vi "Prj2_Main.vi"() -> ()   [LabVIEW 2020]
doc: "Use this template to build a producer/consumer design pattern with events to produce queue items. Use this design pattern instead of the User Interface Event Handler pattern for user interfaces when you want to execute code asynchronously in response to an event without slowing the user interface responsiveness."
uses:
  <vilib>/Instr/_visa.llb/VISA Configure Serial Port (Instr).vi
panel:
  in  "SERVO SPEED [RPS]":dbl
  out "Forward Servo":dbl(knob) scale=0.0..180.0
  out "Reward Servo":dbl(knob) scale=0.0..180.0
  in  "Position":dbl(knob) scale=0.0..180.0
  in  "Manual/Auto":bool
  out "Data Read":string
  in  "Baud rate (9600)":u32=9600
  in  "Write Data":bool
  in  "VISA resource name":refnum<visa-resource-name>
  in  "Close":bool
  in  "Open":bool
  out "Connected":bool
  in  "stop":bool
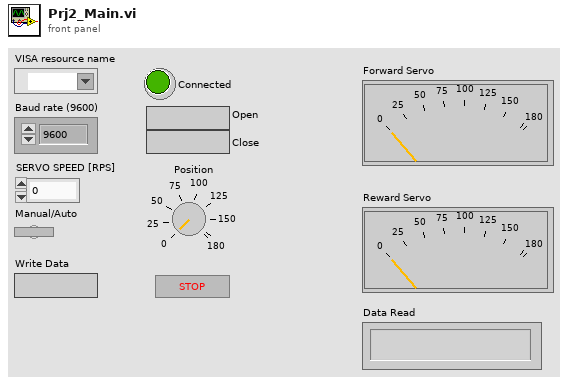
[diagram p1: front panel]
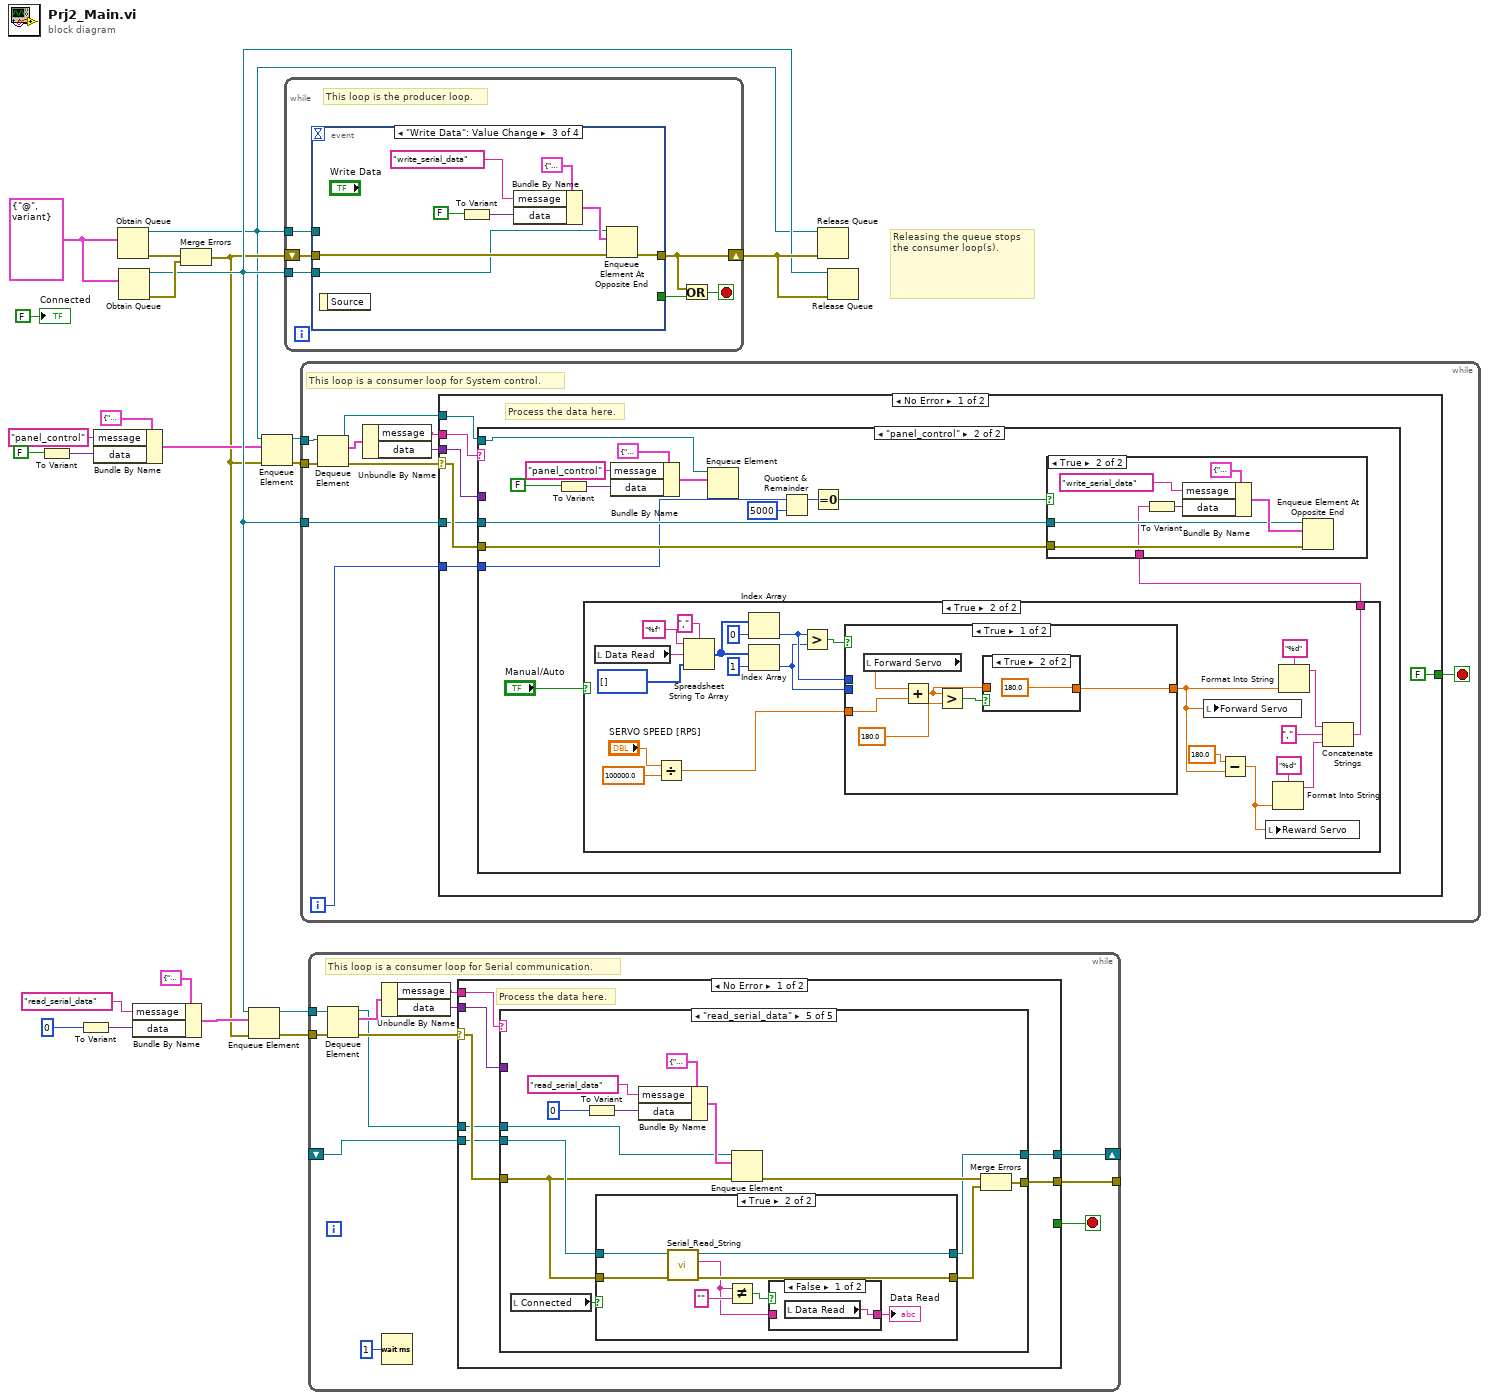
[diagram p0: block diagram]
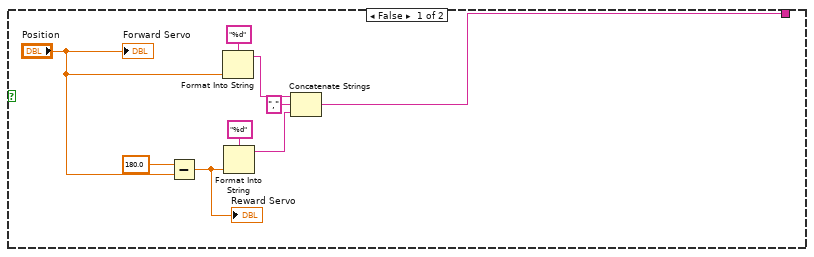
[diagram p3: hidden frame]
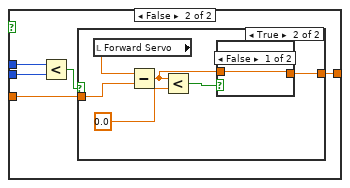
[diagram p5: hidden frame]
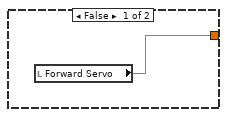
[diagram p6: hidden frame]
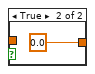
[diagram p7: hidden frame]
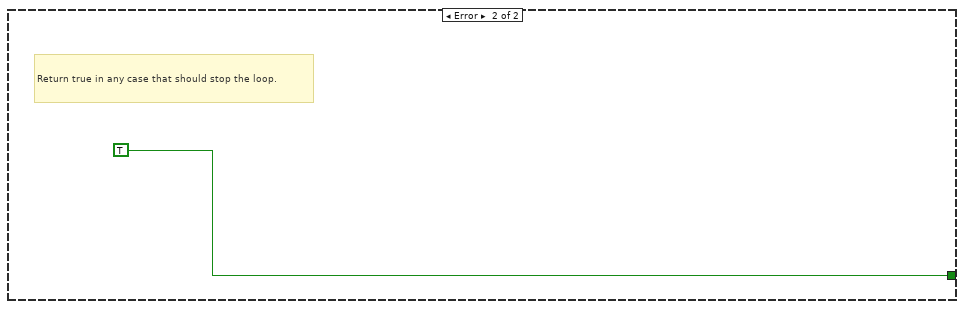
[diagram p9: hidden frame]
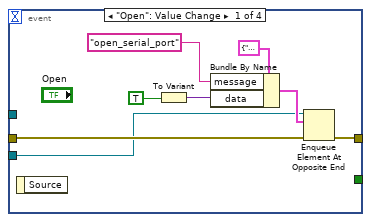
[diagram p10: hidden frame]
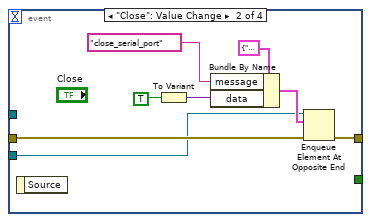
[diagram p11: hidden frame]
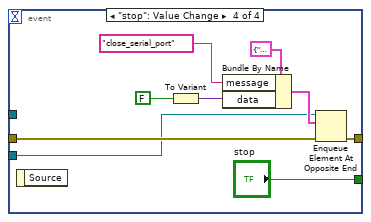
[diagram p12: hidden frame]
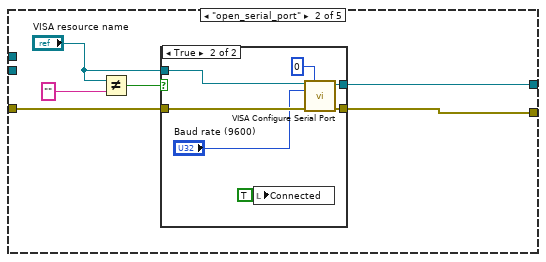
[diagram p14: hidden frame]
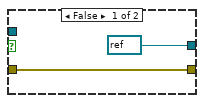
[diagram p15: hidden frame]
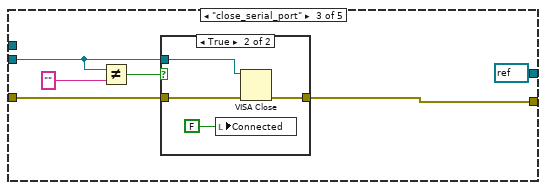
[diagram p16: hidden frame]
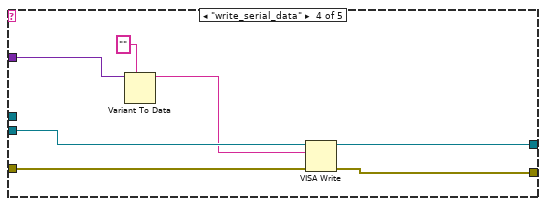
[diagram p18: hidden frame]
diagram:
  w21 = cluster{"message":string, "data":variant} {"message"="@", "data"=variant}
  # "Releasing the queue stops the consumer loop(s)."
  n1 = To Variant(anything=FALSE ("Write Data")) -> (Variant=w9:variant)
  n2 = To Variant(anything=0) -> (Variant=w14:variant)
  n3 = Bundle By Name(cluster=cluster{"message":string, "data":variant} {"message"="@", "data"=variant}, "message"="panel_control", "data"=w9) -> (w8:cluster{"message":string, "data":variant})
  n4 = Obtain Queue(element data type=w21) -> (queue out=w1:refnum<queue>, error out=w20:errorcluster)  [unwired: 4 in, 1 out]
  n5 = Obtain Queue(element data type=w21) -> (queue out=w10:refnum<queue>, error out=w19:errorcluster)  [unwired: 4 in, 1 out]
  n6 = Bundle By Name(cluster=cluster{"message":string, "data":variant} {"message"="@", "data"=variant}, "message"="read_serial_data", "data"=w14) -> (w17:cluster{"message":string, "data":variant})
  n7 = Merge Errors(w20, w19) -> (w3:errorcluster)
  n8 = Enqueue Element(queue=w10, element=w17, error in (no error)=w3) -> (queue out=w11:refnum<queue>, error out=w12:errorcluster)  [unwired: 1 in, 1 out]
  n9 = Enqueue Element(queue=w1, element=w8, error in (no error)=w3) -> (queue out=w2:refnum<queue>, error out=w4:errorcluster)  [unwired: 1 in, 1 out]
  n10 = while {
    shift-right: [w24] -> w18
    shift-left: w3 -> [w27]
    tunnel: w1 -> [w28]
    tunnel: w10 -> [w23]
    stop <- w25 stop-if-true
    # "This loop is the producer loop."
    n11 = event shown="[2] \"Write Data\": Value Change" {
      selector: _ -> [_ _ _ _]
      dyn-events: _ -> [_ _ _ _]
      timeout: _ -> [_ _ _ _]
      tunnel: w28 -> [_ _ _ _]
      tunnel: w27 -> [w32 w40 w48 w56]
      tunnel: [w31 w39 w47 w55] -> w24
      tunnel: [_ _ _ "stop"] -> w26
      tunnel: w23 -> [w30 w38 w46 w54]
      event "Open": Value Change {
        n12 = event-data() -> ()  [unwired: 1 in, 1 out]
        n13 = To Variant(anything=TRUE ("Open")) -> (Variant=w33:variant)
        n14 = Bundle By Name(cluster=cluster{"message":string, "data":variant} {"message"="@", "data"=variant}, "message"="open_serial_port", "data"=w33) -> (w36:cluster{"message":string, "data":variant})
        n15 = Enqueue Element At Opposite End(queue=w30, element=w36, error in (no error)=w32) -> (error out=w31:errorcluster)  [unwired: 1 in, 2 out]
      }
      event "Close": Value Change {
        n16 = event-data() -> ()  [unwired: 1 in, 1 out]
        n17 = To Variant(anything=TRUE ("Close")) -> (Variant=w41:variant)
        n18 = Bundle By Name(cluster=cluster{"message":string, "data":variant} {"message"="@", "data"=variant}, "message"="close_serial_port", "data"=w41) -> (w44:cluster{"message":string, "data":variant})
        n19 = Enqueue Element At Opposite End(queue=w38, element=w44, error in (no error)=w40) -> (error out=w39:errorcluster)  [unwired: 1 in, 2 out]
      }
      event "Write Data": Value Change {
        n20 = event-data() -> ()  [unwired: 1 in, 1 out]
        n21 = To Variant(anything=FALSE ("Write Data")) -> (Variant=w49:variant)
        n22 = Bundle By Name(cluster=cluster{"message":string, "data":variant} {"message"="@", "data"=variant}, "message"="write_serial_data", "data"=w49) -> (w52:cluster{"message":string, "data":variant})
        n23 = Enqueue Element At Opposite End(queue=w46, element=w52, error in (no error)=w48) -> (error out=w47:errorcluster)  [unwired: 1 in, 2 out]
      }
      event "stop": Value Change {
        n24 = event-data() -> ()  [unwired: 1 in, 1 out]
        n25 = To Variant(anything=FALSE ("stop")) -> (Variant=w57:variant)
        n26 = Bundle By Name(cluster=cluster{"message":string, "data":variant} {"message"="@", "data"=variant}, "message"="close_serial_port", "data"=w57) -> (w60:cluster{"message":string, "data":variant})
        n27 = Enqueue Element At Opposite End(queue=w54, element=w60, error in (no error)=w56) -> (error out=w55:errorcluster)  [unwired: 1 in, 2 out]
      }
    }
    n28 = Or(x=w24, y=w26) -> (x .or. y?=w25:bool)
  }
  n29 = while {
    tunnel: w2 -> [w71]
    tunnel: w4 -> [w67]
    tunnel: w10 -> [w64]
    i -> [w63]
    stop <- w69 stop-if-true
    # "This loop is a consumer loop for System control."
    n30 = Dequeue Element(queue=w71, error in (no error)=w67) -> (queue out=w62:refnum<queue>, element=w68:cluster{"message":string, "data":variant}, error out=w70:errorcluster)  [unwired: 1 in, 1 out]
    n31 = Unbundle By Name(w68) -> ("message"=w66:string, "data"=w65:variant)
    n32 = case shown="No Error" w70 {
      selector: w70 -> [w76 _]
      tunnel: [FALSE TRUE] -> w69
      tunnel: w66 -> [w78 _]
      tunnel: w65 -> [w77 _]
      tunnel: w64 -> [w75 _]
      tunnel: w63 -> [w74 _]
      tunnel: w62 -> [w73 _]
      frame No Error {
        # "Process the data here."
        n33 = case shown="\"panel_control\"" w78 {
          tunnel: w77 -> [_ _]
          tunnel: w76 -> [_ w91]
          tunnel: w75 -> [_ w92]
          tunnel: w74 -> [_ w88]
          tunnel: w73 -> [_ w81]
          frame "False", Default {
          }
          frame "panel_control" {
            n34 = To Variant(anything=FALSE ("Write Data")) -> (Variant=w87:variant)
            n35 = case shown="True" "Manual/Auto" {
              tunnel: [w96 w111] -> w79
              frame False {
                n36 = Subtract(x=180.0, y="Position") -> (x-y=w94:dbl)
                "Reward Servo" <- w94
                n37 = Format Into String(format string="%d", "Position") -> (resulting string=w99:string)  [unwired: 2 in, 1 out]
                n38 = Format Into String(format string="%d", w94) -> (resulting string=w97:string)  [unwired: 2 in, 1 out]
                n39 = Concatenate Strings(w99, "," ("string"), w97) -> (w96:string)
                "Forward Servo" <- "Position"
              }
              frame True {
                n40 = local read "Data Read"() -> (w122:string)
                n41 = Divide(x="SERVO SPEED [RPS]", y=100000.0) -> (x/y=w102:dbl)
                n42 = Spreadsheet String To Array(delimiter (Tab)=",", format string="%f", spreadsheet string=w122, array type (2D Dbl)=i32[] [] ("default (0 I32)")) -> (array=w120:i32[])
                n43 = Index Array(array=w120, index=0) -> (element=w109:i32)
                n44 = Index Array(array=w120, index=1) -> (element=w108:i32)
                n45 = Greater?(x=w109, y=w108) -> (0:w117:bool)
                n46 = case shown="True" w117 {
                  tunnel: w102 -> [w129 w136]
                  tunnel: [w124 w135] -> w106
                  tunnel: w109 -> [_ w134]
                  tunnel: w108 -> [_ w133]
                  frame True {
                    n47 = local read "Forward Servo"() -> (w128:dbl)
                    n48 = Add(x=w128, y=w129) -> (x+y=w125:dbl)
                    n49 = Greater?(x=w125, y=180.0) -> (0:w126:bool)
                    n50 = case shown="True" w126 {
                      tunnel: [w130 180.0 ("Horizontal Servo")] -> w124
                      tunnel: w125 -> [w130 _]
                      frame False {
                      }
                      frame True {
                      }
                    }
                  }
                  frame False {
                    n51 = Less?(x=w134, y=w133) -> (x < y?=w132:bool)
                    n52 = case shown="True" w132 {
                      tunnel: w136 -> [_ w143]
                      tunnel: [w137 w138] -> w135
                      frame False {
                        n53 = local read "Forward Servo"() -> (w137:dbl)
                      }
                      frame True {
                        n54 = local read "Forward Servo"() -> (w142:dbl)
                        n55 = Subtract(x=w142, y=w143) -> (x-y=w139:dbl)
                        n56 = Less?(x=w139, y=0.0) -> (x < y?=w140:bool)
                        n57 = case shown="False" w140 {
                          tunnel: [w144 0.0 ("Horizontal Servo")] -> w138
                          tunnel: w139 -> [w144 _]
                          frame False {
                          }
                          frame True {
                          }
                        }
                      }
                    }
                  }
                }
                n58 = local write "Forward Servo"(w106) -> ()
                n59 = Subtract(x=180.0, y=w106) -> (x-y=w105:dbl)
                n60 = local write "Reward Servo"(w105) -> ()
                n61 = Format Into String(format string="%d", w105) -> (resulting string=w112:string)  [unwired: 2 in, 1 out]
                n62 = Format Into String(format string="%d", w106) -> (resulting string=w113:string)  [unwired: 2 in, 1 out]
                n63 = Concatenate Strings(w113, "," ("string"), w112) -> (w111:string)
              }
            }
            n64 = Bundle By Name(cluster=cluster{"message":string, "data":variant} {"message"="@", "data"=variant}, "message"="panel_control", "data"=w87) -> (w86:cluster{"message":string, "data":variant})
            n65 = Enqueue Element(queue=w81, element=w86) -> ()  [unwired: 2 in, 3 out]
            n66 = Quotient & Remainder(x=w88, y=5000) -> (x-y*floor(x/y)=w89:i32)  [unwired: 1 out]
            n67 = Equal To 0?(x=w89) -> (x = 0?=w82:bool)
            n68 = case shown="True" w82 {
              tunnel: w92 -> [_ w148]
              tunnel: w91 -> [_ w147]
              tunnel: w79 -> [_ w146]
              frame False {
              }
              frame True {
                n69 = To Variant(anything=w146) -> (Variant=w149:variant)
                n70 = Bundle By Name(cluster=cluster{"message":string, "data":variant} {"message"="@", "data"=variant}, "message"="write_serial_data", "data"=w149) -> (w152:cluster{"message":string, "data":variant})
                n71 = Enqueue Element At Opposite End(queue=w148, element=w152, error in (no error)=w147) -> ()  [unwired: 1 in, 3 out]
              }
            }
          }
        }
      }
      frame Error {
        # "Return true in any case that should stop the loop."
      }
    }
  }
  n72 = while {
    tunnel: w11 -> [w165]
    tunnel: w12 -> [w161]
    shift-right: [w158] -> _
    shift-left: _ -> [w157]
    tunnel: [w156] -> _
    stop <- w163 stop-if-true
    # "This loop is a consumer loop for Serial communication."
    n73 = Dequeue Element(queue=w165, error in (no error)=w161) -> (queue out=w155:refnum<queue>, element=w162:cluster{"message":string, "data":variant}, error out=w164:errorcluster)  [unwired: 1 in, 1 out]
    n74 = Unbundle By Name(w162) -> ("message"=w160:string, "data"=w159:variant)
    n75 = Wait (ms)(milliseconds to wait=u32 1) -> ()  [unwired: 1 out]
    n76 = case shown="No Error" w164 {
      selector: w164 -> [w170 w233]
      tunnel: [_ TRUE] -> w163
      tunnel: w160 -> [w172 _]
      tunnel: w159 -> [w171 _]
      tunnel: [w169 w234] -> w158
      tunnel: w157 -> [w168 w234]
      tunnel: [w167 w233] -> w156
      tunnel: w155 -> [w166 _]
      frame No Error {
        # "Process the data here."
        n77 = case shown="\"read_serial_data\"" w172 {
          tunnel: w171 -> [_ _ _ w202 _]
          tunnel: w170 -> [w173 w180 w195 w205 w213]
          tunnel: [w174 w176 refnum<visa-resource-name> refnum ("VISA resource name out") w204 w209] -> w169
          tunnel: w168 -> [w174 _ w192 w207 w214]
          tunnel: [w173 w175 w191 w203 w210] -> w167
          tunnel: w166 -> [_ _ _ _ w216]
          frame "False", Default {
          }
          frame "open_serial_port" {
            n78 = Not Equal?(x="VISA resource name", y="") -> (x != y?=w178:bool)
            n79 = case shown="True" w178 {
              tunnel: w180 -> [w181 w188]
              tunnel: "VISA resource name" -> [_ w185]
              tunnel: [refnum<visa-resource-name> refnum ("VISA resource name") w186] -> w176
              tunnel: [w181 w187] -> w175
              frame False {
              }
              frame True {
                n80 = local write "Connected"(TRUE ("Boolean")) -> ()
                n81 = call-poly "VISA Configure Serial Port"("VISA resource name"=w185, "timeout (10sec)"=u32 0, "baud rate (9600)"="Baud rate (9600)", "error in (no error)"=w188) -> ("VISA resource name out"=w186:refnum<visa-resource-name>, "error out"=w187:errorcluster)  [unwired: 10 in]
              }
            }
          }
          frame "close_serial_port" {
            n82 = Not Equal?(x=w192, y="") -> (x != y?=w193:bool)
            n83 = case shown="True" w193 {
              tunnel: w195 -> [w196 w200]
              tunnel: w192 -> [_ w199]
              tunnel: [w196 w197] -> w191
              frame False {
              }
              frame True {
                n84 = local write "Connected"(FALSE ("Boolean")) -> ()
                n85 = VISA Close(VISA resource name=w199, error in (no error)=w200) -> (error out=w197:errorcluster)
              }
            }
          }
          frame "write_serial_data" {
            n86 = Variant To Data(type="", Variant=w202) -> (data=w206:string)  [unwired: 1 in, 1 out]
            n87 = VISA Write(VISA resource name=w207, write buffer=w206, error in (no error)=w205) -> (VISA resource name out=w204:refnum<visa-resource-name>, error out=w203:errorcluster)  [unwired: 1 out]
          }
          frame "read_serial_data" {
            n88 = local read "Connected"() -> (w208:bool)
            n89 = To Variant(anything=0) -> (Variant=w217:variant)
            n90 = case shown="True" w208 {
              tunnel: w214 -> [w222 w228]
              tunnel: w213 -> [w221 w227]
              tunnel: [w221 w230] -> w211
              tunnel: [w222 w229] -> w209
              frame False {
              }
              frame True {
                n91 = call "Serial_Read_String.vi"("error in (no error)"=w227, "VISA Refnum in"=w228) -> ("error out"=w230:errorcluster, "read buffer"=w223:string, "VISA Refnum out"=w229:refnum<visa-resource-name>)  [unwired: 7 in]
                n92 = Not Equal?(x=w223, y="") -> (x != y?=w225:bool)
                n93 = case shown="False" w225 {
                  tunnel: [w231 w232] -> w224
                  tunnel: w223 -> [_ w232]
                  frame False {
                    n94 = local read "Data Read"() -> (w231:string)
                  }
                  frame True {
                  }
                }
                "Data Read" <- w224
              }
            }
            n95 = Bundle By Name(cluster=cluster{"message":string, "data":variant} {"message"="@", "data"=variant}, "message"="read_serial_data", "data"=w217) -> (w220:cluster{"message":string, "data":variant})
            n96 = Enqueue Element(queue=w216, element=w220, error in (no error)=w213) -> (error out=w212:errorcluster)  [unwired: 1 in, 2 out]
            n97 = Merge Errors(w212, w211) -> (w210:errorcluster)
          }
        }
      }
      frame Error {
        # "Return true in any case that should stop the loop."
      }
    }
  }
  n98 = Release Queue(queue=w1, error in (no error)=w18) -> ()  [unwired: 1 in, 3 out]
  n99 = Release Queue(queue=w10, error in (no error)=w18) -> ()  [unwired: 1 in, 3 out]
  "Connected" <- FALSE ("Boolean")
